vi "Random_Index.vi"() -> (0 "Position":cluster{"Row":i32, "Col":i32})   [LabVIEW 2018]
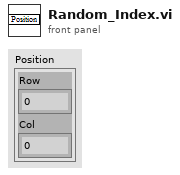
[diagram p1: front panel]
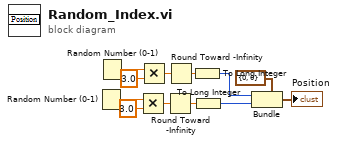
[diagram p0: block diagram]
diagram:
  n1 = Random Number (0-1)() -> (number: 0 to 1=w4:dbl)
  n2 = Random Number (0-1)() -> (number: 0 to 1=w9:dbl)
  n3 = Multiply(x=w4, y=3.0) -> (x*y=w6:dbl)
  n4 = Multiply(x=w9, y=3.0) -> (x*y=w7:dbl)
  n5 = Round Toward -Infinity(1:w6) -> (0:w10:dbl)
  n6 = Round Toward -Infinity(1:w7) -> (0:w2:dbl)
  n7 = To Long Integer(number=w2) -> (32bit integer=w11:i32)
  n8 = To Long Integer(number=w10) -> (32bit integer=w12:i32)
  n9 = Bundle(cluster=cluster{"Row":i32, "Col":i32} {"Row"=0, "Col"=0} ("Position"), "Row"=w11, "Col"=w12) -> (→"Position":cluster{"Row":i32, "Col":i32})
